vi "Simple Edge Counting - Finite Buffered.vi"() -> ()   [LabVIEW 2009]
uses:
  <vilib>/DAQmx/read.llb/DAQmx Read (Counter 1D DBL 1Chan NSamp).vi
  <vilib>/DAQmx/configure/timing.llb/DAQmx Timing (Sample Clock).vi
  <vilib>/DAQmx/create/channels.llb/DAQmx Create Channel (CI-Count Edges).vi
  Program Files/National Instruments/LabVIEW 2009/resource/objmgr/daqmx.rc
panel:
  out "data":dbl[](array[numeric]) format="%0.2f"
  in  "source":tag="/Dev1/PFI9"
  in  "rate":dbl=1000.0 format="%0.2f"
  in  "samples per channel":i32=8
  in  "count direction":i32(ring)=10128 items=["Count Up"=10128, "Count Down"=10124, "Externally Controlled"=10326]
  in  "initial count":u32
  in  "counter":tag="Dev1/ctr0"
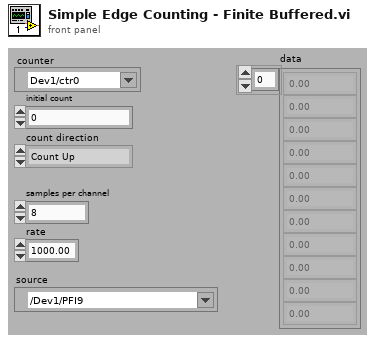
[diagram p1: front panel]
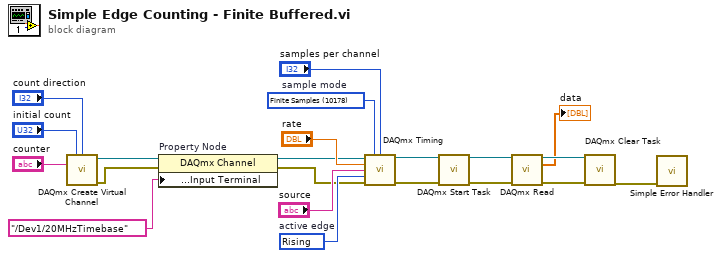
[diagram p0: block diagram]
diagram:
  w6 = 10280 items=["Rising"=10280, "Falling"=10171]  # active edge
  w13 = 10178 items=["Finite Samples"=10178, "Continuous Samples"=10123]  # sample mode
  n1 = call-poly <vilib>:"DAQmx Create Virtual Channel.vi"("initial count"="initial count", "count direction"="count direction", "counter"="counter") -> ("task out"=w5:refnum<k21>, "error out"=w4:errorcluster)  [unwired: 11 in]
  n2 = property on="Property Node" class="DAQmx Channel"(reference=w5, error in=w4, "Counter Input:Count Edges:Input Terminal"=tag "/Dev1/20MHzTimebase" ("CI.CountEdges.Term")) -> (reference out=w2:refnum<k21>, error out=w1:errorcluster)
  n3 = call-poly <vilib>:"DAQmx Timing.vi"("task/channels in"=w2, "sample mode"=w13, "samples per channel"="samples per channel", "rate"="rate", "source"="source", "active edge"=w6, "error in"=w1) -> ("task out"=w11:refnum<k21>, "error out"=w10:errorcluster)  [unwired: 7 in]
  n4 = call <vilib>:"DAQmx Start Task.vi"("task/channels in"=w11, "error in"=w10) -> ("task out"=w18:refnum<k21>, "error out"=w17:errorcluster)  [unwired: 12 in]
  n5 = call-poly <vilib>:"DAQmx Read.vi"("task/channels in"=w18, "error in"=w17) -> ("task out"=w16:refnum<k21>, "data"=→"data":dbl[], "error out"=w15:errorcluster)  [unwired: 11 in]
  n6 = call <vilib>:"DAQmx Clear Task.vi"("task in"=w16, "error in"=w15) -> ("error out"=w14:errorcluster)  [unwired: 13 in]
  n7 = call <vilib>:"Simple Error Handler.vi"("error in (no error)"=w14) -> ()  [unwired: 4 in, 5 out]
